vi "Test Complex Number Add.vi"() -> ()   [LabVIEW 2014]
uses:
  Complex Numbers.lvlib
panel:
  out "Error Out":errorcluster
  in  "Error In":errorcluster
  out "Add":u32
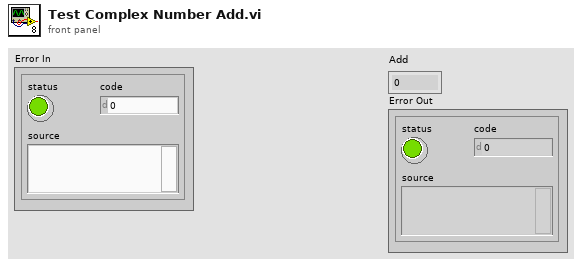
[diagram p1: front panel]
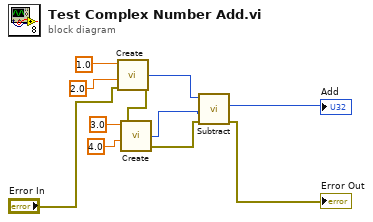
[diagram p0: block diagram]
diagram:
  n1 = call "Create.vi"("Error In"="Error In", "Imag"=2.0 ("Real"), "Real"=1.0) -> ("Error Out"=w8:errorcluster, "Complex"=w5:u32)  [unwired: 2 in]
  n2 = call "Create.vi"("Error In"=w8, "Imag"=4.0 ("Real"), "Real"=3.0) -> ("Error Out"=w3:errorcluster, "Complex"=w4:u32)  [unwired: 2 in]
  n3 = call "Subtract.vi"("Error In"=w3, "Cmpl. B"=w4, "Cmpl. A"=w5) -> ("Error Out"=→"Error Out":errorcluster, "Subtract"=→"Add":u32)  [unwired: 7 in]
